vi "SSC Digital Apply Levels and Timing.vi"(0 "Digital SSC In":T1[](array[typedef]), 5 "Levels Sheet":string, 7 "Timing Sheet":string, 11 "error in":errorcluster) -> (4 "Digital SSC Out":T1[](array[typedef]), 15 "error out":errorcluster)   [LabVIEW 2019]
doc: "Applies digital levels and timing values defined in previously loaded levels and timing sheets to the device(s) connected to the specified pin(s) and pin group(s)."
uses:
  SSC Digital.ctl
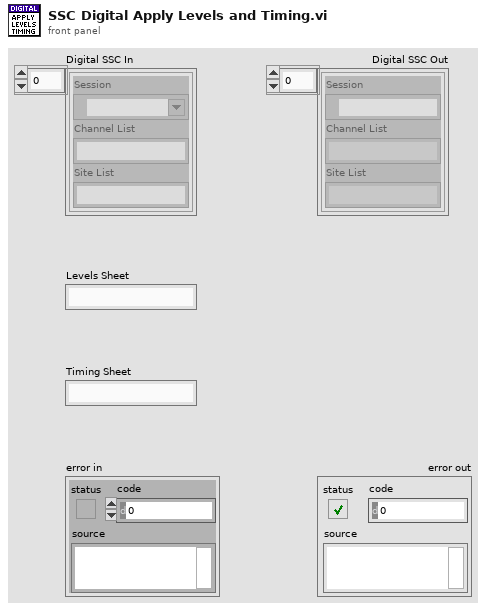
[diagram p1: front panel]
types:
  T1 = typedef "SSC Digital.ctl" = cluster{"Session":refnum<k15>, "Channel List":string, "Site List":string}
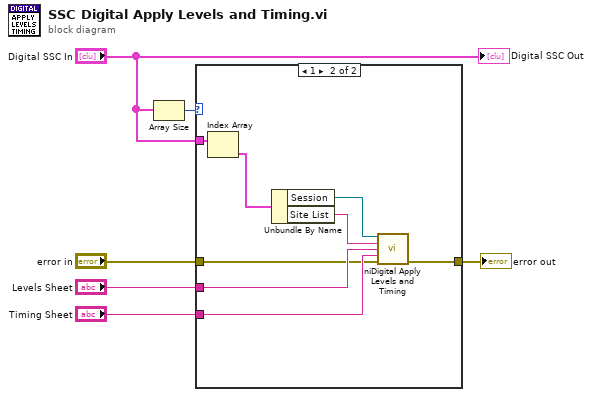
[diagram p0: block diagram]
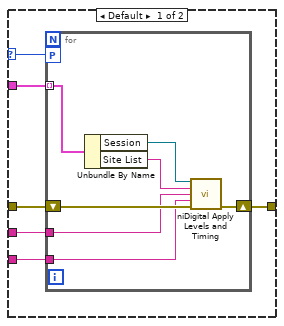
[diagram p2: hidden frame]
diagram:
  n1 = Array Size(array="Digital SSC In") -> (size(s)=w2:i32)
  n2 = case shown="1" w2 {
    selector: w2 -> [w8 _]
    tunnel: "Levels Sheet" -> [w12 w27]
    tunnel: "Timing Sheet" -> [w11 w26]
    tunnel: [w10 w25] -> w4
    tunnel: "error in" -> [w9 w24]
    tunnel: "Digital SSC In" -> [w7 w23]
    frame Default {
      n3 = for {
        workers-P: w8 -> [_]
        tunnel: w12 -> [w17]
        tunnel: w11 -> [w16]
        shift-right: [w18] -> w10
        shift-left: w9 -> [w19]
        tunnel: w7 -> [w15] mode=indexing
        n4 = Unbundle By Name(w15) -> ("Session"=w14:refnum<k15>, "Site List"=w13:string)
        n5 = call <instrlib>:"niDigital Apply Levels and Timing.vi"("instrument handle"=w14, "site list"=w13, "levels sheet"=w17, "timing sheet"=w16, "error in"=w19) -> ("error out"=w18:errorcluster)  [unwired: 9 in, 1 out]
      }
    }
    frame 1 {
      n6 = Index Array(array=w23) -> (element=w20:T1)  [unwired: 1 in]
      n7 = Unbundle By Name(w20) -> ("Session"=w22:refnum<k15>, "Site List"=w21:string)
      n8 = call <instrlib>:"niDigital Apply Levels and Timing.vi"("instrument handle"=w22, "site list"=w21, "levels sheet"=w27, "timing sheet"=w26, "error in"=w24) -> ("error out"=w25:errorcluster)  [unwired: 9 in, 1 out]
    }
  }
  "error out" <- w4
  "Digital SSC Out" <- "Digital SSC In"
